vi "Configure Initial Source Port.vi"(5 "Port (1)":i32=1, 8 "error in (no error)":errorcluster, 10 "Source Port Control State (T: Enable)":bool=TRUE, 11 "VISA resource name":refnum<visa-resource-name>) -> (0 "error out":errorcluster, 3 "VISA resource name out":refnum<visa-resource-name>)   [LabVIEW 2018, in "Agilent ENA Series.lvlib"]
doc: "Configures initial source port."
uses:
  Agilent ENA Series.lvlib
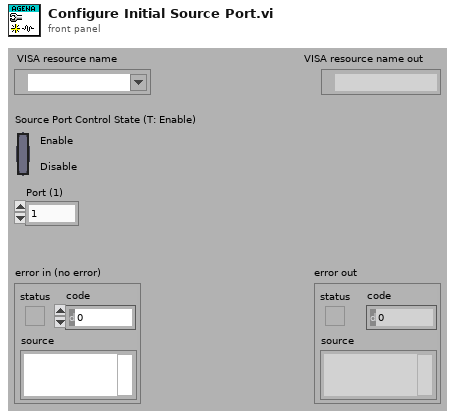
[diagram p1: front panel]
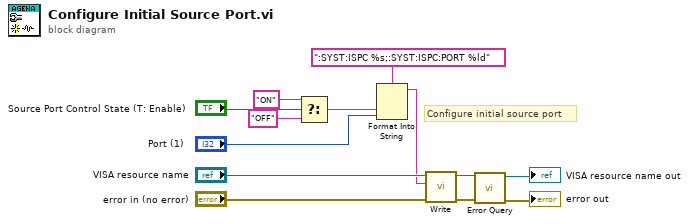
[diagram p0: block diagram]
diagram:
  # "Configure initial source port"
  n1 = Select(t="ON", s="Source Port Control State (T: Enable)", f="OFF") -> (s? t:f=w6:string)
  n2 = Format Into String(format string=":SYST:ISPC %s;:SYST:ISPC:PORT %ld", w6, "Port (1)") -> (resulting string=w10:string)  [unwired: 2 in, 1 out]
  n3 = call "Write.vi"("error in (no error)"="error in (no error)", "String ()"=w10, "VISA resource name"="VISA resource name") -> ("error out"=w3:errorcluster, "VISA resource name out"=w4:refnum<visa-resource-name>)  [unwired: 6 in, 1 out]
  n4 = call "Error Query.vi"("error in (no error)"=w3, "VISA resource name"=w4) -> ("error out"=→"error out":errorcluster, "VISA resource name out"=→"VISA resource name out":refnum<visa-resource-name>)  [unwired: 6 in, 2 out]
